vi "PCert-ConfigPageNF-TellDB.vi"(6 "Timeout":i32=500, 8 "error in (no error)":errorcluster, 9 "Message Body":string, 10 "Message Header":string="Testing", 11 "ERP-ConfigPageNF in":refnum<class "PCert-ConfigPageNF.lvclass">) -> (0 "error out":errorcluster, 3 "ERP-ConfigPageNF out":refnum<class "PCert-ConfigPageNF.lvclass">)   [LabVIEW 2013, in "PCert-ConfigPageNF.lvclass"]
uses:
  PCert-ConfigPageNF.lvclass
  PCert-ConfigPageNF.lvclass/PCert-ConfigPageNF.ctl
  ftw-dataflow/Actor/src/Connector/FTW-ActorConnector.lvclass
panel:
  out "Timed out?":bool
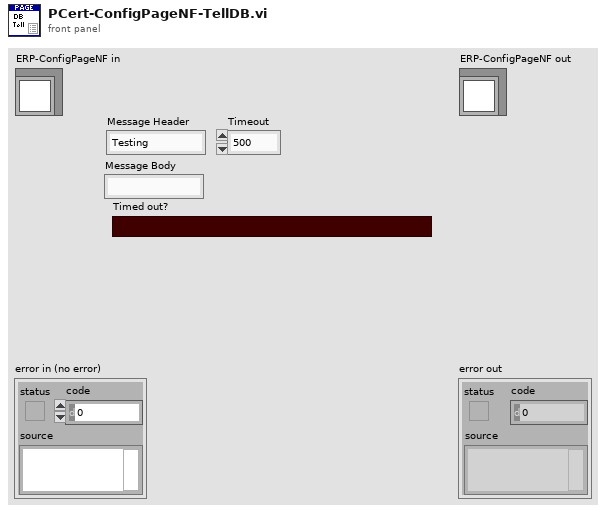
[diagram p1: front panel]
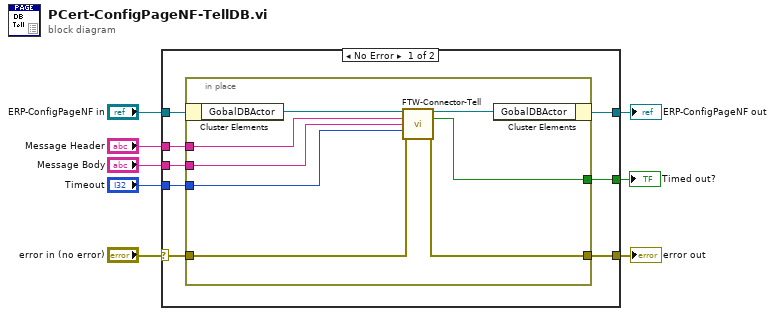
[diagram p0: block diagram]
diagram:
  n1 = case shown="No Error" "error in (no error)" {
    selector: "error in (no error)" -> [w16 w26]
    tunnel: [w15 w26] -> w7
    tunnel: [w13 w25] -> w5
    tunnel: "ERP-ConfigPageNF in" -> [w14 w25]
    tunnel: "Message Header" -> [w12 _]
    tunnel: "Message Body" -> [w11 _]
    tunnel: "Timeout" -> [w10 _]
    tunnel: [w9 _] -> w1
    frame No Error {
      n2 = in-place {
        in-place-border: w16 -> [w22]
        in-place-border: [w21] -> w15
        in-place-border: w12 -> [w20]
        in-place-border: w11 -> [w19]
        in-place-border: w10 -> [w18]
        in-place-border: [w17] -> w9
        n3 = in-place-cluster #1(w14) -> ("GobalDBActor"=w24:refnum<class "FTW-ActorConnector.lvclass">)
        n4 = call "FTW-Connector-Tell.vi"("FTW Actor Connector"=w24, "Message Header"=w20, "Message Body"=w19, "Timeout"=w18, "error in"=w22) -> ("FTW Actor Connector out"=w23:refnum<class "FTW-ActorConnector.lvclass">, "Timed out?"=w17:bool, "error out"=w21:errorcluster)  [unwired: 8 in]
        n5 = in-place-cluster #1("GobalDBActor"=w23) -> (w13:refnum<class "PCert-ConfigPageNF.lvclass">)
      }
    }
    frame Error {
    }
  }
  "error out" <- w7
  "ERP-ConfigPageNF out" <- w5
  "Timed out?" <- w1
